vi "Append Line Breaks to Report.vi"(0 "report in":refnum<class "NI_report.lvclass">, 5 "number of line breaks":u32=1, 11 "error in (no error)":errorcluster) -> (4 "report out":refnum<class "NI_report.lvclass">, 15 "error out":errorcluster)   [LabVIEW 2020, in "NI_ReportGenerationCore.lvlib"]
doc: "Starts a new line in the report."
uses:
  NI_ReportGenerationCore.lvlib
  NI_report.lvclass
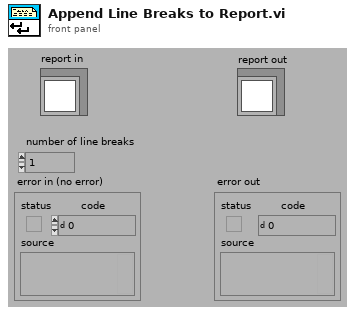
[diagram p1: front panel]
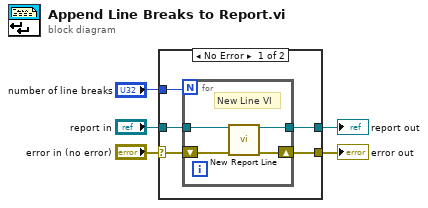
[diagram p0: block diagram]
diagram:
  n1 = case shown="No Error" "error in (no error)" {
    selector: "error in (no error)" -> [w10 w16]
    tunnel: [w9 w15] -> w4
    tunnel: [w8 w16] -> w3
    tunnel: "report in" -> [w7 w15]
    tunnel: "number of line breaks" -> [w6 _]
    frame No Error {
      n2 = for {
        N: w6 -> [_]
        tunnel: w7 -> [w14]
        tunnel: [w13] -> w9
        shift-right: [w11] -> w8
        shift-left: w10 -> [w12]
        # "New Line VI"
        n3 = call-dynamic "New Report Line.vi"("report in"=w14, "error in (no error)"=w12) -> ("report out"=w13:refnum<class "NI_report.lvclass">, "error out"=w11:errorcluster)  [unwired: 12 in]
      }
    }
    frame Error {
    }
  }
  "error out" <- w3
  "report out" <- w4
